vi "Convert Bitpacked U8 DMA.vi"(10 "Channels":i32, 11 "binary array":u8[](array[numeric])) -> (3 "Data":u8[][](array[numeric]))   [LabVIEW 2015, in "FPGA Addon Engine.lvlib"]
uses:
  FPGA Addon Engine.lvlib
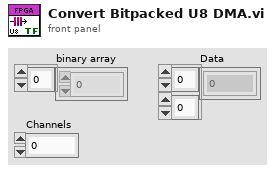
[diagram p1: front panel]
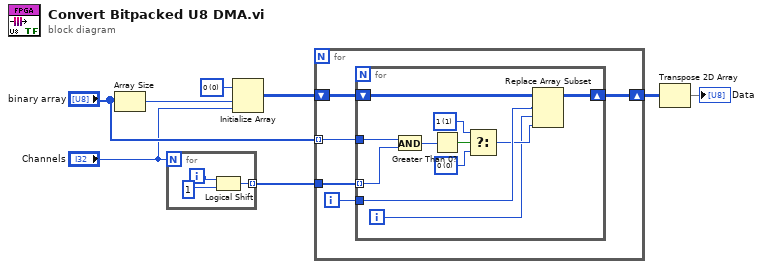
[diagram p0: block diagram]
diagram:
  w3 = u8 0 items=["0", "1", "Z", "L", "H", "X", "T", "V"] ("Digital Values")
  n1 = Array Size(array="binary array") -> (size(s)=w2:i32)
  n2 = for {
    N: "Channels" -> [_]
    tunnel: [w9] -> w1 mode=indexing
    i -> [w10]
    n3 = Logical Shift(y=w10, x=u8 1) -> (x << y=w9:u8)
  }
  n4 = Initialize Array(w3, w2, "Channels") -> (w4:u8[][])
  n5 = for {
    tunnel: "binary array" -> [w16] mode=indexing
    tunnel: w1 -> [w15]
    shift-right: [w12] -> w5
    shift-left: w4 -> [w14]
    i -> [w13]
    n6 = for {
      tunnel: w16 -> [w27]
      tunnel: w15 -> [w26] mode=indexing
      shift-right: [w18] -> w12
      shift-left: w14 -> [w21]
      tunnel: w13 -> [w20]
      i -> [w17]
      w23 = u8 0 items=["0", "1", "Z", "L", "H", "X", "T", "V"] ("Digital Values")
      w22 = u8 1 items=["0", "1", "Z", "L", "H", "X", "T", "V"] ("Digital Values")
      n7 = And(x=w27, y=w26) -> (x .and. y?=w25:u8)
      n8 = Greater Than 0?(x=w25) -> (x > 0?=w24:bool)
      n9 = Select(t=w22, s=w24, f=w23) -> (s? t:f=w19:u8)
      n10 = Replace Array Subset(array=w21, new element=w19, index (row)=w20, index (col)=w17) -> (w18:u8[][])
    }
  }
  n11 = Transpose 2D Array(2D array=w5) -> (transposed array=→"Data":u8[][])
